vi "SSS_V2.1.vi"() -> ()   [LabVIEW 2017]
uses:
  <vilib>/DAQmx/write.llb/DAQmx Write (Analog Wfm 1Chan NSamp).vi
  <vilib>/DAQmx/read.llb/DAQmx Read (Analog 1D Wfm NChan NSamp).vi
  <vilib>/measure/maspectr.llb/FFT Power Spectrum and PSD for 1 Chan.vi
  <vilib>/DAQmx/create/channels.llb/DAQmx Create Channel (AO-Voltage-Basic).vi
  <vilib>/DAQmx/configure/timing.llb/DAQmx Timing (Sample Clock).vi
  <vilib>/DAQmx/miscellaneous.llb/DAQmx Fill In Error Info.vi
  <vilib>/Analysis/3filter.llb/FIR Filter (DBL).vi
  <vilib>/Analysis/NI_AALBase.lvlib
  <vilib>/measure/NI_MAPro.lvlib
panel:
  out "unsigned byte array":u8[][](array[numeric])
  out "숫자형 컨트롤 2":i32
  out "숫자형 컨트롤":i32
  out "배열":i32[](array[numeric])
  out "LED":bool
  in  "STOP":bool
  out "Pack(4byte)":string
  out "크기":i32
  out "Signal Processing Result":waveform(dbl)(graph)
  out "Signal Processing Result 2":waveform(dbl)(graph)
  out "RX.CH1":waveform(dbl)(graph)
  out "RX.CH2":waveform(dbl)(graph)
  out "TX Signal":waveform(dbl)(graph)
  out "TX Spectrum":cluster{"f0":dbl, "df":dbl, "magnitude":dbl[]}(graph)
  in  "포트 번호":u16=6340
  in  "주소":string="30.0.1.228"
  in  "Pulse length(sec)":dbl=0.032 format="%#_6p"
  in  "Stop Frequency(Hz)":dbl=34000.0 format="%#_6p"
  in  "Start Frequency(Hz)":dbl=30000.0 format="%#_6p"
  in  "송신 채널 설정":tag="Dev3/ao1"
  in  "송신 디바이스 이름":tag="Dev3"
  in  "Number of Sample":i32=19200
  in  "RX Time(sec)":dbl=0.2
  in  "수신 디바이스 이름":tag="Dev3"
  in  "수신 채널 설정":tag="Dev3/ai0:1"
  in  "sampling rate":dbl=192000.0 caption="Sampling Frequency" format="%0.2f"
  in  "sample mode":i32(ring)=10123 caption="샘플 모드" items=["유한 샘플"=10178, "연속 샘플"=10123, "하드웨어 타이밍에 의한 단일 포인트"=12522]
  # "송신신호 설정"
  # "디바이스 설정"
  # "TCP 설정"
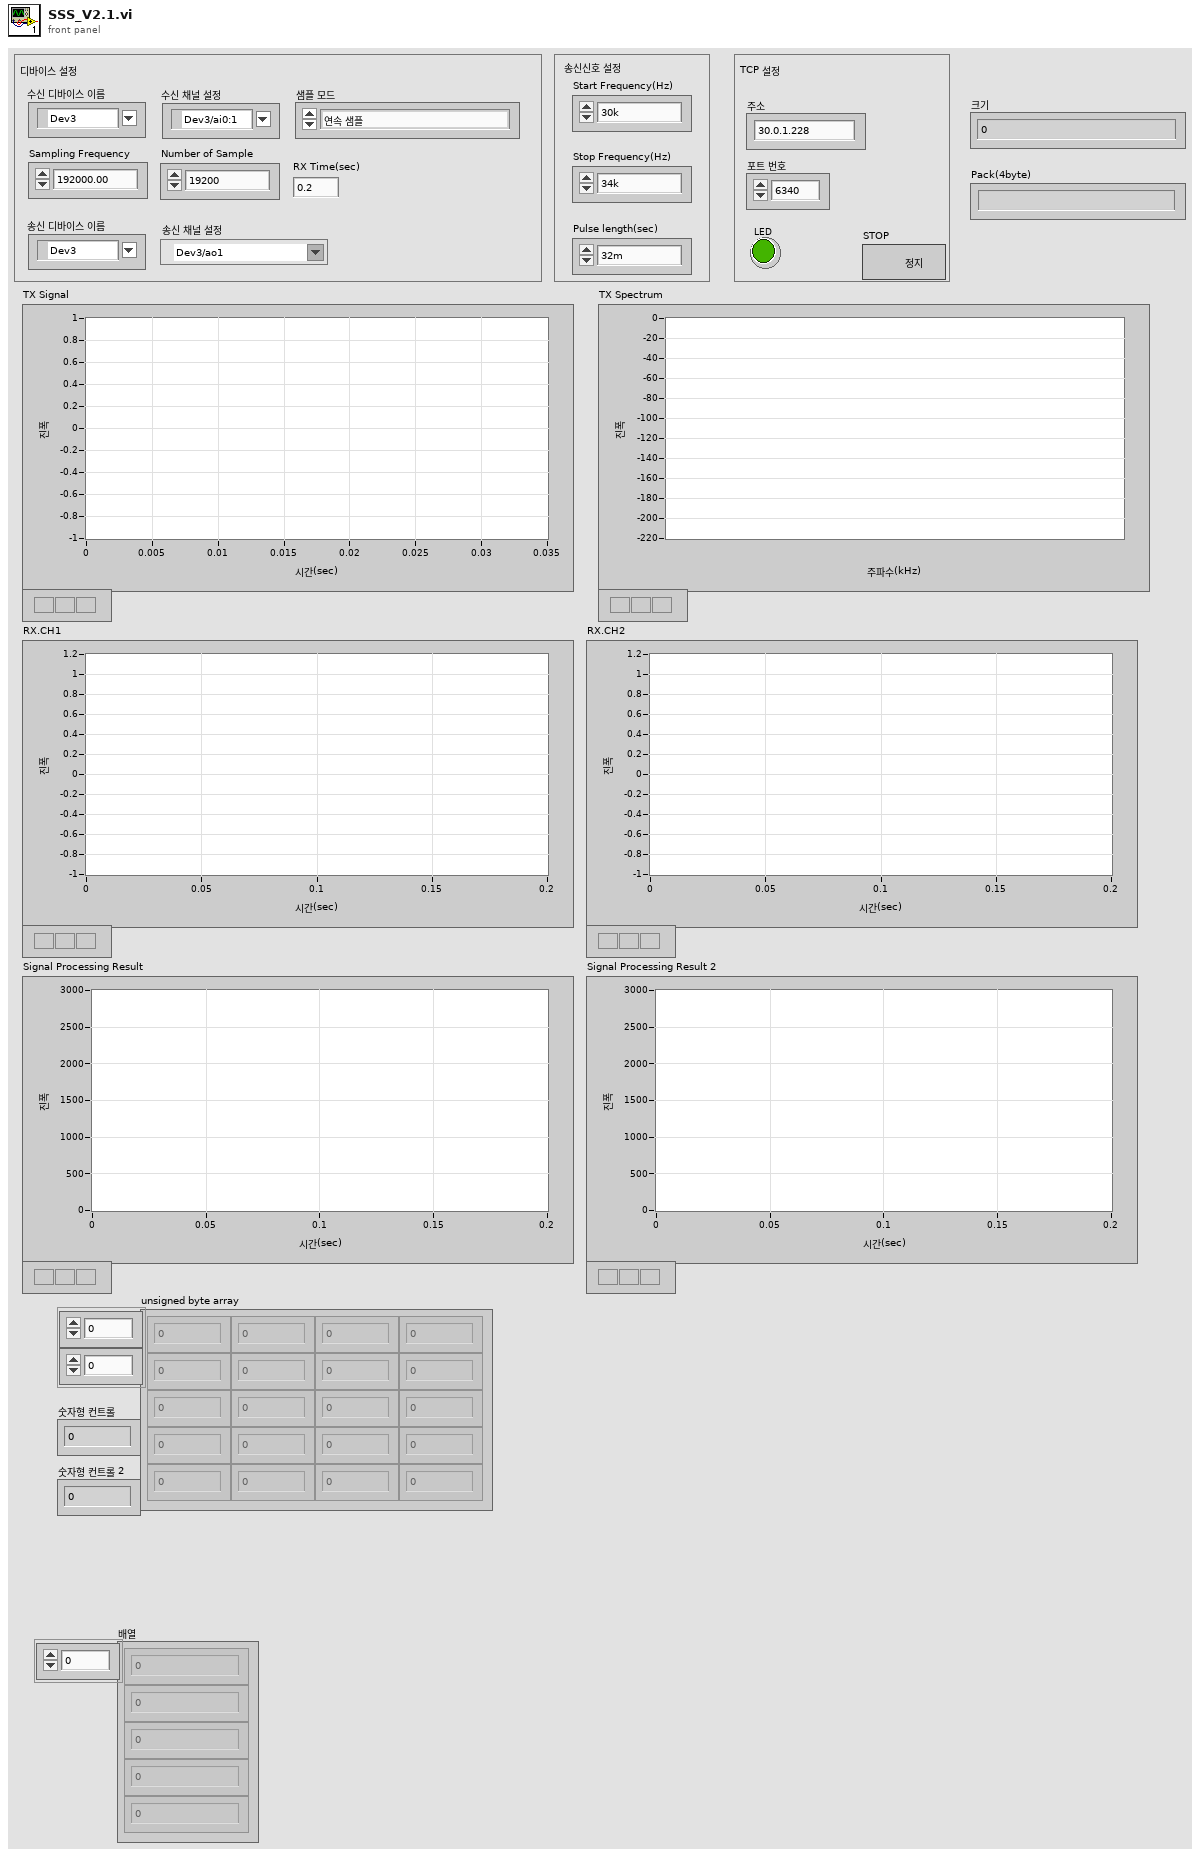
[diagram p1: front panel]
types:
  T1 = enum16{"Standard", "Buffered", "CRLF", "Immediate"}
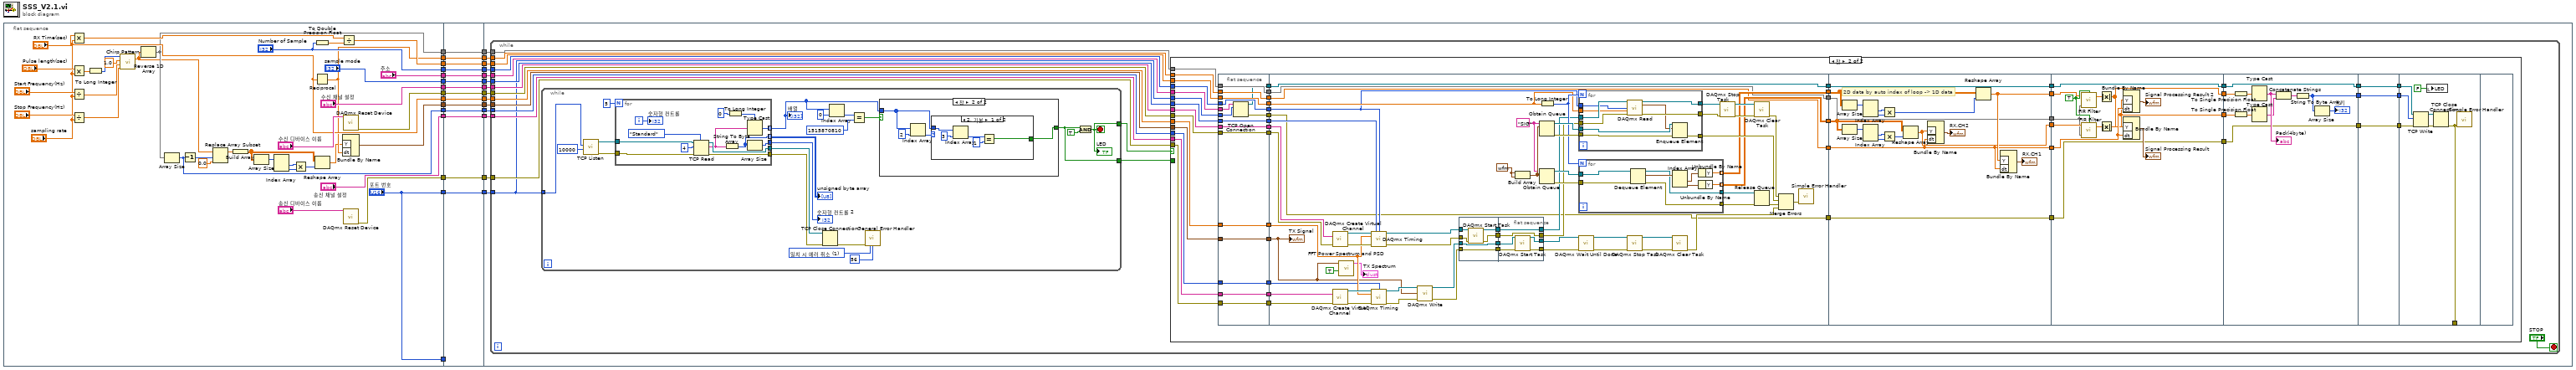
[diagram p0: block diagram]
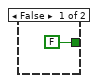
[diagram p3: hidden frame]
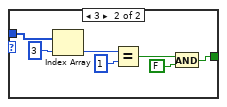
[diagram p4: hidden frame]
diagram:
  n1 = flat-sequence {
    tunnel: ["수신 채널 설정"] -> w29
    tunnel: ["sampling rate"] -> w27
    tunnel: ["송신 채널 설정"] -> w25
    tunnel: ["sample mode"] -> w23
    tunnel: ["Number of Sample"] -> w21
    tunnel: [w53] -> w19
    tunnel: [w52] -> w17
    tunnel: [w45] -> w15
    tunnel: [w46] -> w13
    tunnel: [w44] -> w11
    tunnel: [w43] -> w9
    tunnel: ["포트 번호"] -> w7
    tunnel: ["주소"] -> w5
    tunnel: [w31] -> w3
    tunnel: ["포트 번호"] -> w1
    tunnel: w29 -> [w80]
    tunnel: [w80] -> w28
    tunnel: w27 -> [w79]
    tunnel: [w79] -> w26
    tunnel: w25 -> [w78]
    tunnel: [w78] -> w24
    tunnel: w23 -> [w77]
    tunnel: [w77] -> w22
    tunnel: w21 -> [w76]
    tunnel: [w76] -> w20
    tunnel: w19 -> [w75]
    tunnel: [w75] -> w18
    tunnel: w17 -> [w74]
    tunnel: [w74] -> w16
    tunnel: w15 -> [w73]
    tunnel: [w73] -> w14
    tunnel: w13 -> [w72]
    tunnel: [w72] -> w12
    tunnel: w11 -> [w71]
    tunnel: [w71] -> w10
    tunnel: w9 -> [w70]
    tunnel: [w70] -> w8
    tunnel: w7 -> [w69]
    tunnel: [w69] -> w6
    tunnel: w5 -> [w68]
    tunnel: [w68] -> w4
    tunnel: w3 -> [w67]
    tunnel: [w67] -> w2
    tunnel: w1 -> [_]
    tunnel: w28 -> [w85]
    tunnel: w26 -> [w84]
    tunnel: w24 -> [w88]
    tunnel: w22 -> [w83]
    tunnel: w20 -> [w82]
    tunnel: w18 -> [w86]
    tunnel: w16 -> [w89]
    tunnel: w14 -> [w94]
    tunnel: w12 -> [w81]
    tunnel: w10 -> [w90]
    tunnel: w8 -> [w93]
    tunnel: w6 -> [w92]
    tunnel: w4 -> [w91]
    tunnel: w2 -> [w87]
    frame #0 {
      n2 = Multiply(x="RX Time(sec)", y="sampling rate") -> (x*y=w50:dbl)
      n3 = Multiply(x="Pulse length(sec)", y="sampling rate") -> (x*y=w65:dbl)
      n4 = Divide(x="Start Frequency(Hz)", y="sampling rate") -> (x/y=w62:dbl)
      n5 = Divide(x="Stop Frequency(Hz)", y="sampling rate") -> (x/y=w59:dbl)
      n6 = To Long Integer(number=w65) -> (32bit integer=w64:i32)
      n7 = call <vilib>:"Chirp Pattern.vi"("f2"=w59, "f1"=w62, "amplitude"=1.0, "samples"=w64) -> ("Chirp Pattern"=w38:dbl[])  [unwired: 1 out]
      n8 = Reverse 1D Array(array=w38) -> (reversed array=w43:dbl[])
      n9 = Array Size(array=w43) -> (size(s)=w31:i32)
      n10 = Decrement(x=w31) -> (x-1=w41:i32)
      n11 = Replace Array Subset(array=w38, new element=0.0 ("새 원소/부분배열"), index=w41) -> (w39:dbl[])
      n12 = Build Array(w39) -> (w33:dbl[][])
      n13 = Array Size(array=w33) -> (size(s)=w34:i32[])
      n14 = Index Array(array=w34) -> (element #1=w36:i32, element #2=w35:i32)  [unwired: 2 in]
      n15 = Multiply(x=w36, y=w35) -> (x*y=w37:i32)
      n16 = To Double Precision Float(number="Number of Sample") -> (double precision float=w51:dbl)
      n17 = Reciprocal(x="sampling rate") -> (1/x=w45:dbl)
      n18 = Reshape Array(w33, w37) -> (w32:dbl[])
      n19 = Divide(x=w50, y=w51) -> (x/y=w46:dbl)
      n20 = Bundle By Name("Y"=w32, "dt"=w45) -> (w44:waveform(dbl))  [unwired: 1 in]
      n21 = call <vilib>:"DAQmx Reset Device.vi"("device in"="수신 디바이스 이름") -> ("error out"=w53:errorcluster)  [unwired: 1 in, 13 out]
      n22 = call <vilib>:"DAQmx Reset Device.vi"("device in"="송신 디바이스 이름") -> ("error out"=w52:errorcluster)  [unwired: 1 in, 13 out]
    }
    frame #1 {
    }
    frame #2 {
      n23 = while {
        tunnel: w85 -> [w111]
        tunnel: w88 -> [w110]
        tunnel: w84 -> [w109]
        tunnel: w83 -> [w108]
        tunnel: w82 -> [w103]
        tunnel: w86 -> [w107]
        tunnel: w89 -> [w106]
        tunnel: w90 -> [w105]
        tunnel: w81 -> [w104]
        tunnel: w94 -> [w102]
        tunnel: w93 -> [w101]
        tunnel: w92 -> [w98]
        tunnel: w91 -> [w100]
        tunnel: w87 -> [w99]
        stop <- "STOP" stop-if-true
        n24 = while {
          tunnel: w98 -> [w326]
          tunnel: [w325] -> w97
          tunnel: [w323] -> w96
          stop <- w325 stop-if-true
          w321 = 1 items=["예외 없음", "일치 시 에러 취소", "일치 시 에러 설정"] ("[exception action] (none:0)")
          n25 = call <vilib>:"TCP Listen.vi"("timeout ms (wait forever: -1)"=10000, "port"=w326) -> ("error out"=w338:errorcluster, "connection ID"=w339:refnum<k5>)  [unwired: 5 in, 3 out]
          n26 = for {
            N: 5 -> [_]
            tunnel: w339 -> [w369]
            tunnel: w338 -> [w368]
            tunnel: [w367] -> w337
            tunnel: [w361] -> w336
            tunnel: [w363] -> w334 mode=indexing
            tunnel: [w362] -> w333
            tunnel: [w357] -> w328 mode=indexing
            i -> [w364]
            n27 = TCP Read(connection ID=w369, bytes to read=4 ("읽을 바이트"), error in (no error)=w368, 7:T1."Standard" ("모드(standard)")) -> (connection ID out=w367:refnum<k5>, data out=w358:string, error out=w361:errorcluster)  [unwired: 1 out]
            n28 = String To Byte Array(string=w358) -> (unsigned byte array=w363:u8[])
            n29 = To Long Integer(number=0 ("숫자")) -> (32bit integer=w360:i32)
            n30 = Type Cast(type=w360, x=w358) -> (*(type *) &x=w357:i32)
            n31 = Array Size(array=w363) -> (size(s)=w362:i32)
            "숫자형 컨트롤" <- w364
          }
          "unsigned byte array" <- w334
          "숫자형 컨트롤 2" <- w333
          "배열" <- w328
          n32 = TCP Close Connection(connection ID=w337, error in (no error)=w336) -> (error out=w322:errorcluster)  [unwired: 2 out]
          n33 = Index Array(array=w328, index=0 ("인덱스")) -> (element=w330:i32)
          n34 = Equal?(x=w330, y=1515870810) -> (x = y?=w329:bool)
          n35 = call <vilib>:"General Error Handler.vi"("error in (no error)"=w322, "[exception action] (none:0)"=w321, "[exception code]"=56) -> ()  [unwired: 8 in, 5 out]
          n36 = case shown="참" w329 {
            tunnel: w328 -> [_ w342]
            tunnel: [FALSE w341] -> w323
            frame False {
            }
            frame True {
              n37 = Index Array(array=w342, index=2 ("인덱스")) -> (element=w343:i32)
              n38 = case shown="2, 기본" w343 {
                tunnel: w342 -> [w349 w356]
                tunnel: [w345 w350] -> w341
                frame 2, Default {
                  n39 = Index Array(array=w349, index=3 ("인덱스")) -> (element=w347:i32)
                  n40 = Equal?(x=w347, y=1) -> (x = y?=w345:bool)
                }
                frame 3 {
                  n41 = Index Array(array=w356, index=3 ("인덱스")) -> (element=w354:i32)
                  n42 = Equal?(x=w354, y=1) -> (x = y?=w352:bool)
                  n43 = And(x=w352, y=FALSE) -> (x .and. y?=w350:bool)
                }
              }
            }
          }
          n44 = And(x=w323, y=TRUE) -> (x .and. y?=w325:bool)
          "LED" <- w325
        }
        n45 = case shown="참" w97 {
          tunnel: w111 -> [_ w125]
          tunnel: w110 -> [_ w124]
          tunnel: w109 -> [_ w123]
          tunnel: w108 -> [_ w122]
          tunnel: w107 -> [_ w121]
          tunnel: w106 -> [_ w120]
          tunnel: w105 -> [_ w119]
          tunnel: w104 -> [_ w118]
          tunnel: w103 -> [_ w117]
          tunnel: w102 -> [_ w116]
          tunnel: w101 -> [_ w115]
          tunnel: w100 -> [_ w114]
          tunnel: w99 -> [_ w113]
          tunnel: w98 -> [_ w112]
          tunnel: w96 -> [_ _]
          frame False {
          }
          frame True {
            n46 = flat-sequence {
              tunnel: w115 -> [w167]
              tunnel: w116 -> [w168]
              tunnel: w117 -> [w169]
              tunnel: w118 -> [w170]
              tunnel: w119 -> [w171]
              tunnel: w120 -> [w172]
              tunnel: w121 -> [w173]
              tunnel: w122 -> [w174]
              tunnel: w123 -> [w175]
              tunnel: w124 -> [w176]
              tunnel: w125 -> [w177]
              tunnel: [w177] -> w161
              tunnel: [w176] -> w160
              tunnel: [w175] -> w159
              tunnel: [w174] -> w158
              tunnel: [w173] -> w157
              tunnel: [w172] -> w156
              tunnel: [w171] -> w155
              tunnel: [w170] -> w154
              tunnel: [w169] -> w153
              tunnel: [w168] -> w152
              tunnel: [w167] -> w151
              tunnel: w112 -> [w166]
              tunnel: w114 -> [w165]
              tunnel: [w164] -> w150
              tunnel: [w163] -> w149
              tunnel: w113 -> [w162]
              tunnel: [w162] -> w148
              tunnel: [w190] -> w147
              tunnel: [w189] -> w146
              tunnel: [w188] -> w145
              tunnel: [w187] -> w144
              tunnel: w161 -> [w232]
              tunnel: w160 -> [w229]
              tunnel: w159 -> [w226]
              tunnel: w158 -> [w225]
              tunnel: w157 -> [w224]
              tunnel: w156 -> [w223]
              tunnel: w155 -> [w183]
              tunnel: w154 -> [w192]
              tunnel: w153 -> [w191]
              tunnel: w152 -> [w188]
              tunnel: w151 -> [w187]
              tunnel: [w185] -> w143
              tunnel: w150 -> [w185]
              tunnel: [w184] -> w142
              tunnel: w149 -> [w184]
              tunnel: w148 -> [w182]
              tunnel: w147 -> [w275]
              tunnel: w146 -> [w274]
              tunnel: w145 -> [w270]
              tunnel: [w273] -> w141
              tunnel: [w272] -> w140
              tunnel: [w271] -> w139
              tunnel: w144 -> [w271]
              tunnel: [w270] -> w138
              tunnel: [w269] -> w137
              tunnel: w143 -> [w269]
              tunnel: [w268] -> w136
              tunnel: w142 -> [w268]
              tunnel: w141 -> [w295]
              tunnel: w140 -> [w294]
              tunnel: w139 -> [w292]
              tunnel: w138 -> [w291]
              tunnel: [w290] -> w135
              tunnel: [w288] -> w134
              tunnel: [w287] -> w133
              tunnel: w137 -> [w287]
              tunnel: [w286] -> w132
              tunnel: w136 -> [w286]
              tunnel: w135 -> [w308]
              tunnel: w134 -> [w306]
              tunnel: [w301] -> w131
              tunnel: [w299] -> w130
              tunnel: [w300] -> w129
              tunnel: w133 -> [w300]
              tunnel: w132 -> [w299]
              tunnel: w131 -> [w312]
              tunnel: [w312] -> w126
              tunnel: w130 -> [w311]
              tunnel: [w311] -> w127
              tunnel: w129 -> [w310]
              tunnel: [w310] -> w128
              tunnel: [w317] -> _
              tunnel: w128 -> [w314]
              tunnel: w127 -> [w315]
              tunnel: w126 -> [w316]
              frame #0 {
                n47 = TCP Open Connection(address=w165, remote port or service name=w166) -> (connection ID=w163:refnum<k5>, error out=w164:errorcluster)  [unwired: 3 in]
              }
              frame #1 {
                w198 = "SIG" ("이름(이름없음)")
                w201 = waveform(dbl) {"t0"=timestamp(0 s since 1904-01-01), "dt"=1.0, "Y"=[]} ("Waveform")
                n48 = call-poly <vilib>:"DAQmx Create Virtual Channel.vi"("physical channels"=w232, "error in"=w224) -> ("task out"=w231:refnum<k21>, "error out"=w230:errorcluster)  [unwired: 7 in, 5 out]
                n49 = call-poly <vilib>:"DAQmx Create Virtual Channel.vi"("physical channels"=w229, "error in"=w223) -> ("task out"=w228:refnum<k21>, "error out"=w227:errorcluster)  [unwired: 7 in, 5 out]
                n50 = call-poly <vilib>:"FFT Power Spectrum and PSD.vi"("dB On (F)"=TRUE, "time signal"=w183) -> ("Power Spectrum / PSD"=→"TX Spectrum":cluster{"f0":dbl, "df":dbl, "magnitude":dbl[]})  [unwired: 6 in, 3 out]
                n51 = call-poly <vilib>:"DAQmx Timing.vi"("task/channels in"=w231, "sample mode"=w225, "samples per channel"=w191, "rate"=w226, "error in"=w230) -> ("task out"=w217:refnum<k21>, "error out"=w218:errorcluster)  [unwired: 2 in, 7 out]
                n52 = call-poly <vilib>:"DAQmx Timing.vi"("task/channels in"=w228, "samples per channel"=w182, "rate"=w226, "error in"=w227) -> ("task out"=w222:refnum<k21>, "error out"=w221:errorcluster)  [unwired: 3 in, 7 out]
                n53 = call-poly <vilib>:"DAQmx Write.vi"("task/channels in"=w222, "data"=w183, "error in"=w221) -> ("task out"=w216:refnum<k21>, "error out"=w215:errorcluster)  [unwired: 10 in, 1 out]
                n54 = flat-sequence {
                  tunnel: w218 -> [w261]
                  tunnel: [w260] -> w236
                  tunnel: [w259] -> w235
                  tunnel: w217 -> [w258]
                  tunnel: w215 -> [w257]
                  tunnel: [w257] -> w234
                  tunnel: w216 -> [w256]
                  tunnel: [w256] -> w233
                  tunnel: w236 -> [w267]
                  tunnel: [w267] -> w193
                  tunnel: [w266] -> w194
                  tunnel: w235 -> [w266]
                  tunnel: w234 -> [w265]
                  tunnel: w233 -> [w264]
                  tunnel: [w263] -> w181
                  tunnel: [w262] -> w178
                  frame #0 {
                    n55 = call <vilib>:"DAQmx Start Task.vi"("task/channels in"=w258, "error in"=w261) -> ("task out"=w259:refnum<k21>, "error out"=w260:errorcluster)  [unwired: 12 in]
                  }
                  frame #1 {
                    n56 = call <vilib>:"DAQmx Start Task.vi"("task/channels in"=w264, "error in"=w265) -> ("task out"=w263:refnum<k21>, "error out"=w262:errorcluster)  [unwired: 12 in]
                  }
                }
                n57 = Build Array(w201, w201) -> (w200:waveform(dbl)[])
                n58 = To Long Integer(number=w192) -> (32bit integer=w199:i32)
                n59 = Obtain Queue(name (unnamed)=w198, element data type=w200) -> (queue out=w210:refnum<queue>, error out=w209:errorcluster)  [unwired: 3 in, 1 out]
                n60 = Obtain Queue(name (unnamed)=w198, element data type=w200) -> (queue out=w204:refnum<queue>, error out=w203:errorcluster)  [unwired: 3 in, 1 out]
                n61 = for {
                  N: w199 -> [_]
                  tunnel: w210 -> [w255]
                  tunnel: w209 -> [w254]
                  tunnel: [w253] -> w207
                  tunnel: [w252] -> w206
                  tunnel: [w251] -> w205
                  tunnel: w194 -> [w249]
                  tunnel: w193 -> [w248]
                  tunnel: w191 -> [w247]
                  tunnel: w192 -> [w246]
                  n62 = call-poly <vilib>:"DAQmx Read.vi"("task/channels in"=w249, "number of samples per channel"=w247, "timeout"=w246, "error in"=w248) -> ("task out"=w252:refnum<k21>, "data"=w250:waveform(dbl)[], "error out"=w251:errorcluster)  [unwired: 9 out]
                  n63 = Enqueue Element(queue=w255, element=w250, error in (no error)=w254) -> (error out=w253:errorcluster)  [unwired: 1 in, 2 out]
                }
                n64 = for {
                  N: w199 -> [_]
                  tunnel: w204 -> [w245]
                  tunnel: w203 -> [w244]
                  tunnel: [w243] -> w197
                  tunnel: [w241] -> w195
                  tunnel: [w238] -> w190 mode=indexing
                  tunnel: [w239] -> w189 mode=indexing
                  n65 = Dequeue Element(queue=w245, error in (no error)=w244) -> (queue out=w241:refnum<queue>, element=w242:waveform(dbl)[], error out=w243:errorcluster)  [unwired: 1 in, 1 out]
                  n66 = Index Array(array=w242) -> (element #1=w240:waveform(dbl), element #2=w237:waveform(dbl))  [unwired: 2 in]
                  n67 = Unbundle By Name(w240) -> ("Y"=w238:dbl[])
                  n68 = Unbundle By Name(w237) -> ("Y"=w239:dbl[])
                }
                n69 = call <vilib>:"DAQmx Wait Until Done.vi"("task/channels in"=w181, "error in"=w178) -> ("task out"=w180:refnum<k21>, "error out"=w179:errorcluster)  [unwired: 12 in]
                n70 = call <vilib>:"DAQmx Stop Task.vi"("task/channels in"=w180, "error in"=w179) -> ("task out"=w214:refnum<k21>, "error out"=w213:errorcluster)  [unwired: 12 in]
                n71 = call <vilib>:"DAQmx Clear Task.vi"("task in"=w214, "error in"=w213) -> ("error out"=w186:errorcluster)  [unwired: 13 in]
                n72 = call <vilib>:"DAQmx Stop Task.vi"("task/channels in"=w206, "error in"=w205) -> ("task out"=w211:refnum<k21>, "error out"=w212:errorcluster)  [unwired: 12 out]
                n73 = call <vilib>:"DAQmx Clear Task.vi"("task in"=w211, "error in"=w212) -> ("error out"=w208:errorcluster)  [unwired: 13 out]
                n74 = Release Queue(queue=w195, error in (no error)=w197) -> (error out=w196:errorcluster)  [unwired: 3 out]
                n75 = Merge Errors(w208, w207, w196, w186) -> (w202:errorcluster)
                n76 = call <vilib>:"Simple Error Handler.vi"("error in (no error)"=w202) -> ()  [unwired: 4 in, 5 out]
                "TX Signal" <- w183
              }
              frame #2 {
                # "2D data by auto index of loop -> 1D data"
                n77 = Array Size(array=w275) -> (size(s)=w282:i32[])
                n78 = Array Size(array=w274) -> (size(s)=w278:i32[])
                n79 = Index Array(array=w282) -> (element #1=w284:i32, element #2=w283:i32)  [unwired: 2 in]
                n80 = Index Array(array=w278) -> (element #1=w280:i32, element #2=w279:i32)  [unwired: 2 in]
                n81 = Multiply(x=w284, y=w283) -> (x*y=w285:i32)
                n82 = Multiply(x=w280, y=w279) -> (x*y=w281:i32)
                n83 = Reshape Array(w274, w281) -> (w272:dbl[])
                n84 = Bundle By Name("Y"=w272, "dt"=w270) -> (→"RX.CH2":waveform(dbl))  [unwired: 1 in]
                n85 = Reshape Array(w275, w285) -> (w273:dbl[])
                n86 = Bundle By Name("Y"=w273, "dt"=w270) -> (→"RX.CH1":waveform(dbl))  [unwired: 1 in]
              }
              frame #3 {
                w297 = TRUE ("init/cont (init:F)")
                n87 = call-poly <vilib>:"FIR Filter.vi"("init/cont (init:F)"=w297, "FIR Coefficients"=w292, "X"=w295) -> ("Filtered X"=w296:dbl[])  [unwired: 1 in, 1 out]
                n88 = call-poly <vilib>:"FIR Filter.vi"("init/cont (init:F)"=w297, "FIR Coefficients"=w292, "X"=w294) -> ("Filtered X"=w293:dbl[])  [unwired: 1 in, 1 out]
                n89 = Absolute Value(x=w296) -> (abs(x)=w290:dbl[])
                n90 = Absolute Value(x=w293) -> (abs(x)=w288:dbl[])
                n91 = Bundle By Name("Y"=w288, "dt"=w291) -> (→"Signal Processing Result 2":waveform(dbl))  [unwired: 1 in]
                n92 = Bundle By Name("Y"=w290, "dt"=w291) -> (→"Signal Processing Result":waveform(dbl))  [unwired: 1 in]
              }
              frame #4 {
                n93 = To Single Precision Float(number=w308) -> (single precision float=w309:sgl[])
                n94 = To Single Precision Float(number=w306) -> (single precision float=w307:sgl[])
                n95 = Type Cast(x=w309) -> (*(type *) &x=w305:string)  [unwired: 1 in]
                "Pack(4byte)" <- w305
                n96 = Type Cast(x=w307) -> (*(type *) &x=w304:string)  [unwired: 1 in]
                n97 = Concatenate Strings(w305, w304) -> (w303:string)
                n98 = String To Byte Array(string=w303) -> (unsigned byte array=w301:u8[])
                n99 = Array Size(array=w301) -> (size(s)=→"크기":i32)
              }
              frame #5 {
              }
              frame #6 {
                n100 = TCP Write(connection ID=w315, data in=w316, error in (no error)=w314) -> (connection ID out=w318:refnum<k5>, error out=w319:errorcluster)  [unwired: 1 in, 1 out]
                n101 = local write "LED"(FALSE) -> ()
                n102 = TCP Close Connection(connection ID=w318, error in (no error)=w319) -> (error out=w317:errorcluster)  [unwired: 1 in, 1 out]
                n103 = call <vilib>:"Simple Error Handler.vi"("error in (no error)"=w317) -> ()  [unwired: 4 in, 5 out]
              }
              frame #7 {
              }
            }
          }
        }
      }
    }
  }
